vi "Rename File.vi"(8 "error in (no error)":errorcluster, 10 "New Filename":string, 11 "Old File Path":path) -> (0 "error out":errorcluster, 2 "Success?":bool)   [LabVIEW 2013]
uses:
  kernel32.dll 
panel:
  # "The Old Filename must be the complete path to the\nfile to be renamed, and the new filename should \njust be the new name of the file (without extension)"
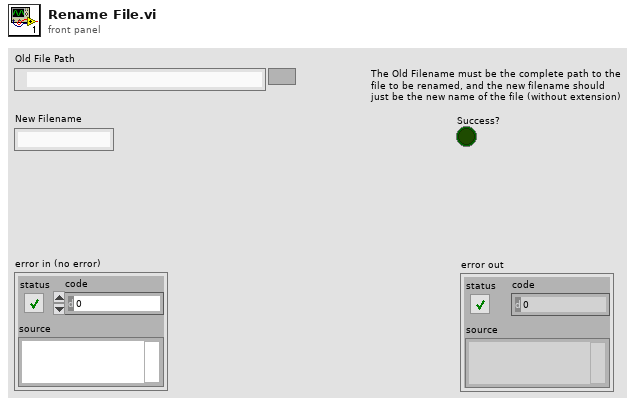
[diagram p1: front panel]
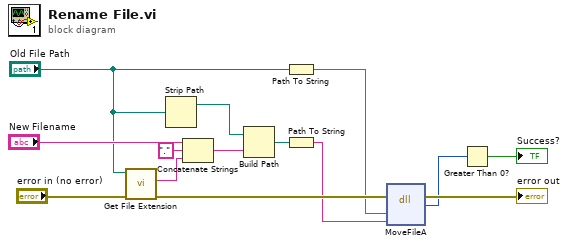
[diagram p0: block diagram]
diagram:
  n1 = call <vilib>:"Get File Extension.vi"("error in (no error)"="error in (no error)", "file"="Old File Path") -> ("error out"=w10:errorcluster, "lowercase file extension"=w2:string)  [unwired: 6 in, 2 out]
  n2 = Strip Path(path="Old File Path") -> (stripped path=w7:path)  [unwired: 1 out]
  n3 = Concatenate Strings("New Filename", "." ("string"), w2) -> (w8:string)
  n4 = Build Path(base path=w7, name or relative path=w8) -> (appended path=w6:path)
  n5 = Path To String(path="Old File Path") -> (string=w5:string)
  n6 = Path To String(path=w6) -> (string=w4:string)
  n7 = dll-call lib="kernel32.dll " fn="MoveFileA"(error in=w10, "arg1"=w5, "arg2"=w4) -> (error out=→"error out":errorcluster, "return type"=w13:i32)  [unwired: 4 in, 1 out]
  n8 = Greater Than 0?(x=w13) -> (x > 0?=→"Success?":bool)
